vi "AB_Log_Build_Preview.vi"(6 "destination path":path, 8 "error in (no error)":errorcluster, 10 "Visible files":path[](array[path]), 11 "All files":path[](array[path])) -> (0 "error out":errorcluster)   [LabVIEW 2020]
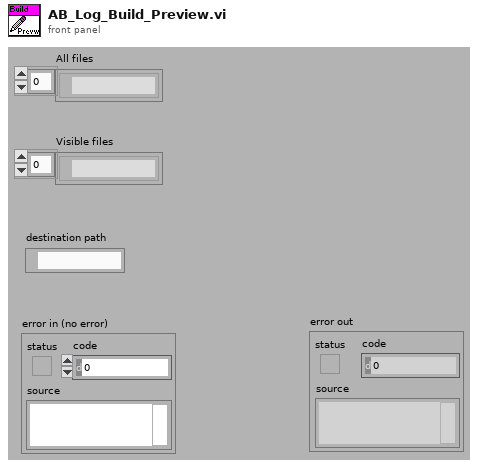
[diagram p1: front panel]
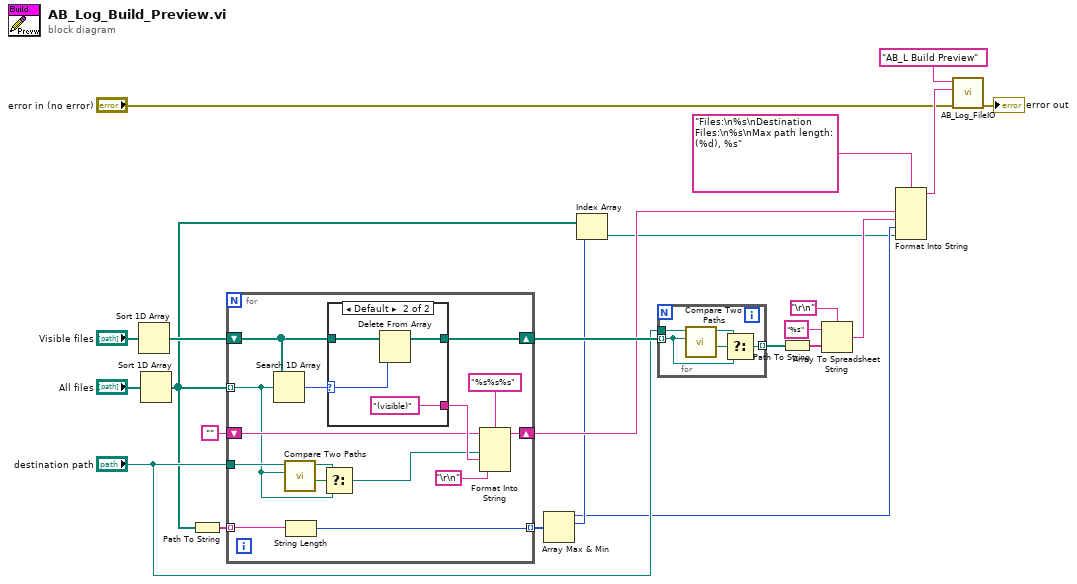
[diagram p0: block diagram]
diagram:
  n1 = Sort 1D Array(array="Visible files") -> (sorted array=w7:path[])
  n2 = Sort 1D Array(array="All files") -> (sorted array=w4:path[])
  n3 = Path To String(path=w4) -> (string=w6:string[])
  n4 = for {
    shift-right: [w36] -> w13
    shift-left: w7 -> [w37]
    tunnel: w4 -> [w27] mode=indexing
    shift-right: [w32] -> w10
    shift-left: "" -> [w31]
    tunnel: "destination path" -> [w30]
    tunnel: w6 -> [w25] mode=indexing
    tunnel: [w24] -> w5 mode=indexing
    n5 = Search 1D Array(1D array=w37, element=w27) -> (index of element=w38:i32)  [unwired: 1 in]
    n6 = call <vilib>:"Compare Two Paths.vi"("Path 2"=w27, "Path 1"=w30) -> ("Path 2 Relative to Path 1?"=w29:bool, "Relative Path from 1 to 2"=w28:path)  [unwired: 6 in, 2 out]
    n7 = String Length(string=w25) -> (length=w24:i32)
    n8 = Select(t=w28, s=w29, f=w27) -> (s? t:f=w26:path)
    n9 = case shown="Default" w38 {
      selector: w38 -> [_ w41]
      tunnel: [_ "(visible)" ("format string")] -> w35
      tunnel: w37 -> [w39 w43]
      tunnel: [w39 w42] -> w36
      frame -1 {
      }
      frame Default {
        n10 = Delete From Array(array=w43, index=w41) -> (array with subset deleted=w42:path[])  [unwired: 1 in, 1 out]
      }
    }
    n11 = Format Into String(format string="%s%s%s", initial string=w31, w26, w35, "\r\n") -> (resulting string=w32:string)  [unwired: 1 in, 1 out]
  }
  n12 = Array Max & Min(array=w5) -> (max value=w2:i32, max index (indices)=w3:i32)  [unwired: 2 out]
  n13 = Index Array(array=w4, index=w3) -> (element=w1:path)
  n14 = for {
    tunnel: w13 -> [w46] mode=indexing
    tunnel: [w45] -> w12 mode=indexing
    tunnel: "destination path" -> [w44]
    n15 = call <vilib>:"Compare Two Paths.vi"("Path 2"=w46, "Path 1"=w44) -> ("Path 2 Relative to Path 1?"=w47:bool, "Relative Path from 1 to 2"=w48:path)  [unwired: 6 in, 2 out]
    n16 = Select(t=w48, s=w47, f=w46) -> (s? t:f=w45:path)
  }
  n17 = Path To String(path=w12) -> (string=w17:string[])
  n18 = Array To Spreadsheet String(delimiter (Tab)="\r\n", array=w17, 3:"%s" ("format string")) -> (spreadsheet string=w14:string)
  n19 = Format Into String(format string="Files:\n%s\nDestination Files:\n%s\nMax path length: (%d), %s", w10, w14, w2, w1) -> (resulting string=w22:string)  [unwired: 2 in, 1 out]
  n20 = call <vilib>:"AB_Log_FileIO.vi"("error in (no error)"="error in (no error)", "data"=w22, "newSection"="AB_L Build Preview" ("data")) -> ("error out"=→"error out":errorcluster)  [unwired: 8 in]
